vi "标样核查.vi"(11 "标样核查配置":T1={"数据保存间隔"=1.0, "水温标样值"=0.0, "pH标样值"=0.0, "溶解氧标样值"=0.0, "电导率标样值"=0.0, "浊度标样值"=0.0}) -> ()   [LabVIEW 2016, in "斯坦道多参数.lvlib"]
panel:
  out "运行状态":u16(ring) items=["空闲", "水样测试", "标样核查"]
  out "seconds since 1Jan1904":timestamp
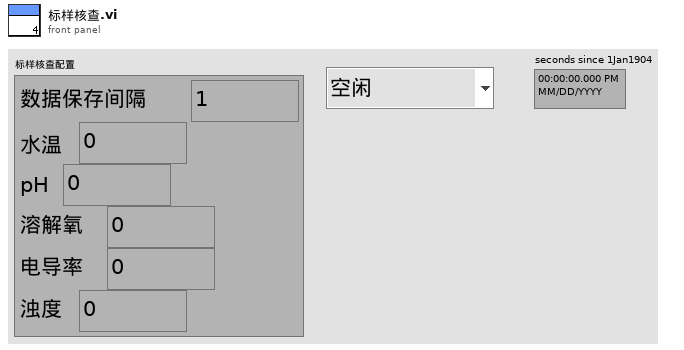
[diagram p1: front panel]
types:
  T1 = cluster{"数据保存间隔":dbl, "水温标样值":dbl, "pH标样值":dbl, "溶解氧标样值":dbl, "电导率标样值":dbl, "浊度标样值":dbl}
  T2 = cluster{"因子编码":string, "单位":string, "标样参考值":sgl, "水样数据时间":timestamp, "水样实测值":sgl, "水样数据标识":string, "探头温度":sgl}
  T3 = typedef "LVDateTimeRec.ctl" = cluster{"秒数的小数部分":dbl, "秒":i32, "分":i32, "时":i32, "日":i32, "月":i32, "年":i32, "天数（周）":i32, "天数（年）":i32, "DST":i32}
  T4 = cluster{"温度测量值":sgl, "DO%":sgl, "DOmg/L":sgl, "温度偏移修正值":sgl}
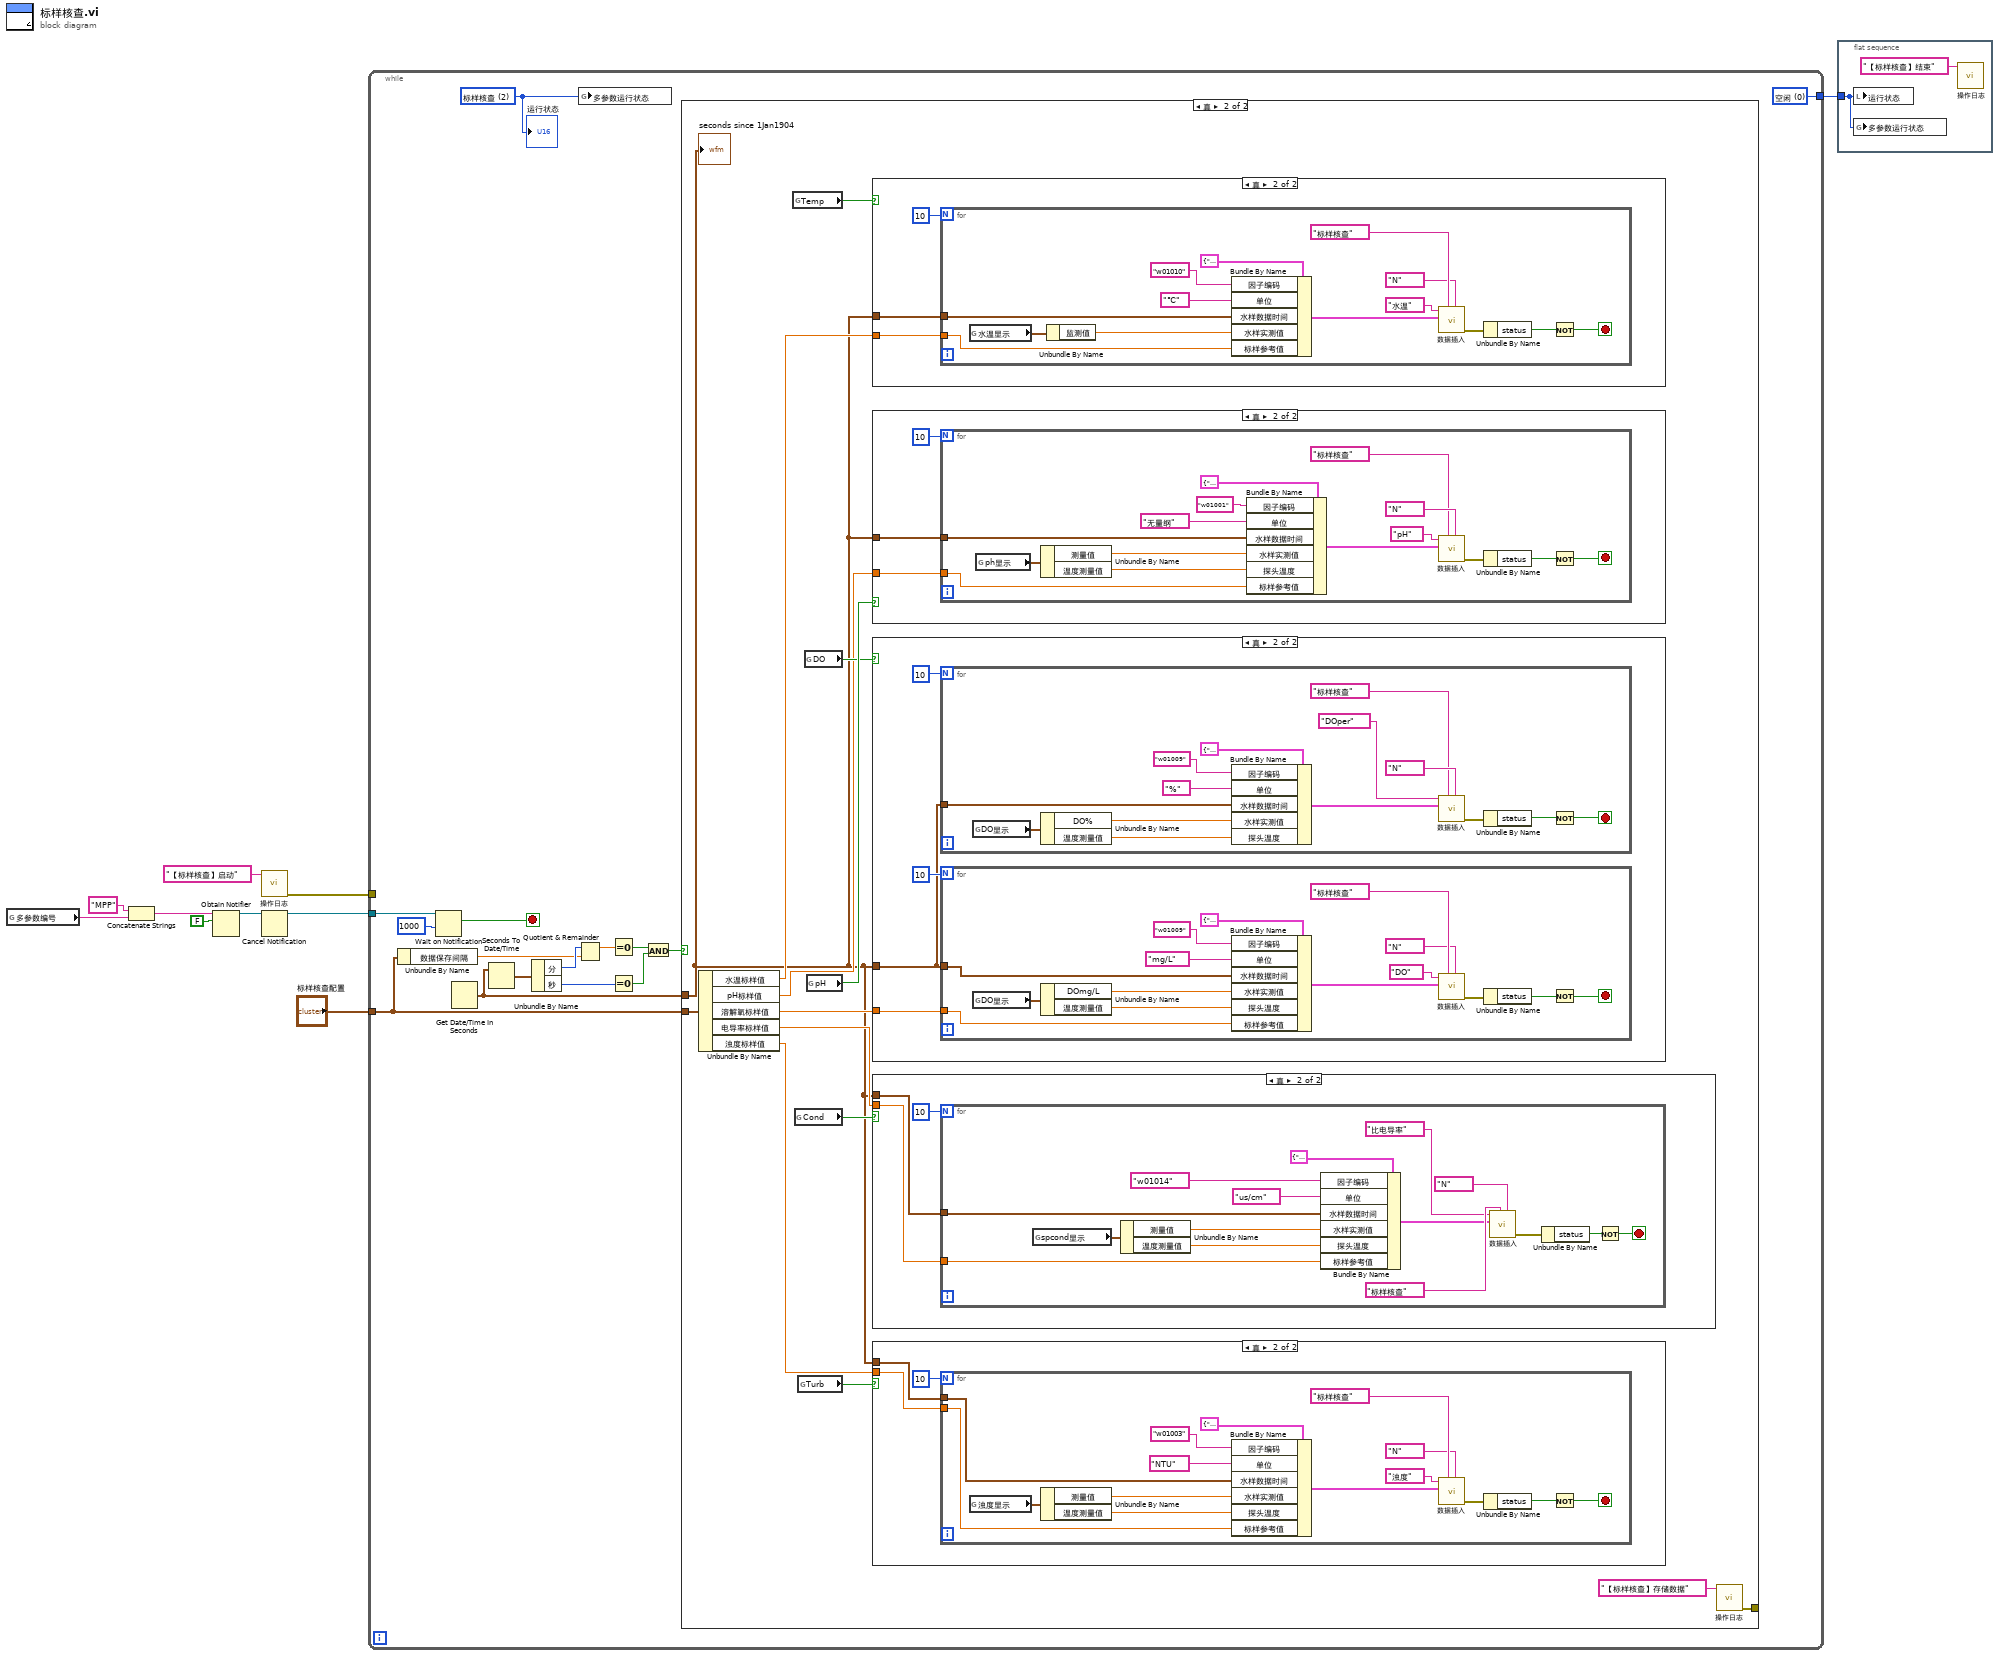
[diagram p0: block diagram]
diagram:
  n1 = global read "多参数全局变量.vi" "多参数编号"() -> (w3:string)
  n2 = Concatenate Strings("MPP" ("名称（未命名）"), w3) -> (w4:string)
  n3 = Obtain Notifier(name (unnamed)=w4, notification data type=FALSE) -> (notifier out=w7:refnum<notifier>)  [unwired: 2 in, 2 out]
  n4 = call "操作日志.vi"("日志信息"="【标样核查】启动") -> ("error out"=w1:errorcluster)  [unwired: 10 in]
  n5 = Cancel Notification(0:w7) -> (8:w6:refnum<notifier>)  [unwired: 1 in, 2 out]
  n6 = while {
    tunnel: "标样核查配置" -> [w21]
    tunnel: [w15] -> w5
    tunnel: w6 -> [w14]
    tunnel: w1 -> [_]
    stop <- w12 stop-if-true
    w15 = u16 0 items=["空闲", "水样测试", "标样核查"] ("多参数运行状态")
    w11 = u16 2 items=["空闲", "水样测试", "标样核查"] ("多参数运行状态")
    n7 = Unbundle By Name(w21) -> ("数据保存间隔"=w19:dbl)
    n8 = Wait on Notification(notifier=w14, timeout in ms (-1)=1000 ("超时毫秒(-1)")) -> (notification=w12:bool)  [unwired: 2 in, 3 out]
    n9 = Get Date/Time In Seconds() -> (seconds since 1Jan1904=w16:timestamp)
    n10 = Seconds To Date/Time(time stamp (now)=w16) -> (date time rec=w25:T3)  [unwired: 1 in]
    n11 = Unbundle By Name(w25) -> ("分"=w20:i32, "秒"=w24:i32)
    n12 = Quotient & Remainder(x=w20, y=w19) -> (x-y*floor(x/y)=w18:dbl)  [unwired: 1 out]
    n13 = global write "多参数全局变量.vi" "多参数运行状态"(w11) -> ()
    n14 = Equal To 0?(x=w18) -> (x = 0?=w17:bool)
    n15 = Equal To 0?(x=w24) -> (x = 0?=w23:bool)
    n16 = And(x=w17, y=w23) -> (x .and. y?=w22:bool)
    n17 = case shown="真" w22 {
      tunnel: w21 -> [_ w34]
      tunnel: w16 -> [_ w26]
      tunnel: [_ w27] -> _
      frame False {
      }
      frame True {
        n18 = Unbundle By Name(w34) -> ("水温标样值"=w33:dbl, "pH标样值"=w32:dbl, "溶解氧标样值"=w31:dbl, "电导率标样值"=w30:dbl, "浊度标样值"=w29:dbl)
        n19 = global read "断电保存变量.vi" "Temp"() -> (w39:bool)
        n20 = global read "断电保存变量.vi" "Cond"() -> (w36:bool)
        n21 = global read "断电保存变量.vi" "Turb"() -> (w35:bool)
        n22 = global read "断电保存变量.vi" "DO"() -> (w37:bool)
        n23 = global read "断电保存变量.vi" "pH"() -> (w38:bool)
        n24 = case shown="真" w39 {
          tunnel: w33 -> [_ w129]
          tunnel: w26 -> [_ w128]
          frame False {
          }
          frame True {
            n25 = for {
              N: 10 -> [_]
              tunnel: w129 -> [w136]
              tunnel: w128 -> [w133]
              stop <- w130 stop-if-true
              n26 = global read "多参数全局变量.vi" "水温显示"() -> (w135:cluster{"CH":u16, "监测值":dbl, "温度偏移修正值":sgl})
              n27 = Unbundle By Name(w135) -> ("监测值"=w134:dbl)
              n28 = Bundle By Name(cluster=T2 {"因子编码"="w01003", "单位"="无量纲", "标样参考值"=0.0, "水样数据时间"=timestamp(0 s since 1904-01-01), "水样实测值"=0.0, "水样数据标识"="N", "探头温度"=0.0} ("data in"), "因子编码"="w01010", "单位"="℃", "水样数据时间"=w133, "水样实测值"=w134, "标样参考值"=w136) -> (w142:T2)
              n29 = call "数据插入.vi"("数据标记表"="N", "测量模式"="标样核查", "data in"=w142, "table输入"="水温") -> ("error out"=w132:errorcluster)  [unwired: 7 in]
              n30 = Unbundle By Name(w132) -> ("status"=w131:bool)
              n31 = Not(x=w131) -> (.not. x?=w130:bool)
            }
          }
        }
        n32 = case shown="真" w38 {
          tunnel: w32 -> [_ w111]
          tunnel: w26 -> [_ w109]
          frame False {
          }
          frame True {
            n33 = for {
              N: 10 -> [_]
              tunnel: w111 -> [w119]
              tunnel: w109 -> [w112]
              stop <- w113 stop-if-true
              n34 = global read "多参数全局变量.vi" "ph显示"() -> (w118:cluster{"温度测量值":sgl, "测量值":sgl, "温度偏移修正值":sgl})
              n35 = Unbundle By Name(w118) -> ("测量值"=w117:sgl, "温度测量值"=w116:sgl)
              n36 = Bundle By Name(cluster=T2 {"因子编码"="w01003", "单位"="无量纲", "标样参考值"=0.0, "水样数据时间"=timestamp(0 s since 1904-01-01), "水样实测值"=0.0, "水样数据标识"="N", "探头温度"=0.0} ("data in"), "因子编码"="w01001", "单位"="无量纲", "水样数据时间"=w112, "水样实测值"=w117, "探头温度"=w116, "标样参考值"=w119) -> (w124:T2)
              n37 = call "数据插入.vi"("数据标记表"="N", "测量模式"="标样核查", "data in"=w124, "table输入"="pH") -> ("error out"=w115:errorcluster)  [unwired: 7 in]
              n38 = Unbundle By Name(w115) -> ("status"=w114:bool)
              n39 = Not(x=w114) -> (.not. x?=w113:bool)
            }
          }
        }
        n40 = case shown="真" w37 {
          tunnel: w31 -> [_ w79]
          tunnel: w26 -> [_ w76]
          frame False {
          }
          frame True {
            n41 = for {
              N: 10 -> [_]
              tunnel: w76 -> [w80]
              stop <- w81 stop-if-true
              n42 = global read "多参数全局变量.vi" "DO显示"() -> (w84:T4)
              n43 = Unbundle By Name(w84) -> ("DO%"=w88:sgl, "温度测量值"=w86:sgl)
              n44 = Bundle By Name(cluster=T2 {"因子编码"="w01003", "单位"="无量纲", "标样参考值"=0.0, "水样数据时间"=timestamp(0 s since 1904-01-01), "水样实测值"=0.0, "水样数据标识"="N", "探头温度"=0.0} ("data in"), "因子编码"="w01009", "单位"="%", "水样数据时间"=w80, "水样实测值"=w88, "探头温度"=w86) -> (w85:T2)
              n45 = call "数据插入.vi"("数据标记表"="N", "测量模式"="标样核查", "data in"=w85, "table输入"="DOper") -> ("error out"=w83:errorcluster)  [unwired: 7 in]
              n46 = Unbundle By Name(w83) -> ("status"=w82:bool)
              n47 = Not(x=w82) -> (.not. x?=w81:bool)
            }
            n48 = for {
              N: 10 -> [_]
              tunnel: w79 -> [w99]
              tunnel: w76 -> [w94]
              stop <- w95 stop-if-true
              n49 = global read "多参数全局变量.vi" "DO显示"() -> (w98:T4)
              n50 = Unbundle By Name(w98) -> ("DOmg/L"=w106:sgl, "温度测量值"=w108:sgl)
              n51 = Bundle By Name(cluster=T2 {"因子编码"="w01003", "单位"="无量纲", "标样参考值"=0.0, "水样数据时间"=timestamp(0 s since 1904-01-01), "水样实测值"=0.0, "水样数据标识"="N", "探头温度"=0.0} ("data in"), "因子编码"="w01009", "单位"="mg/L", "水样数据时间"=w94, "水样实测值"=w106, "探头温度"=w108, "标样参考值"=w99) -> (w105:T2)
              n52 = call "数据插入.vi"("数据标记表"="N", "测量模式"="标样核查", "data in"=w105, "table输入"="DO") -> ("error out"=w97:errorcluster)  [unwired: 7 in]
              n53 = Unbundle By Name(w97) -> ("status"=w96:bool)
              n54 = Not(x=w96) -> (.not. x?=w95:bool)
            }
          }
        }
        n55 = case shown="真" w36 {
          tunnel: w30 -> [_ w60]
          tunnel: w26 -> [_ w58]
          frame False {
          }
          frame True {
            n56 = for {
              N: 10 -> [_]
              tunnel: w60 -> [w68]
              tunnel: w58 -> [w61]
              stop <- w62 stop-if-true
              n57 = global read "多参数全局变量.vi" "spcond显示"() -> (w67:cluster{"温度测量值":sgl, "测量值":sgl, "温度偏移修正值":sgl})
              n58 = Unbundle By Name(w67) -> ("测量值"=w66:sgl, "温度测量值"=w65:sgl)
              n59 = Bundle By Name(cluster=T2 {"因子编码"="w01003", "单位"="无量纲", "标样参考值"=0.0, "水样数据时间"=timestamp(0 s since 1904-01-01), "水样实测值"=0.0, "水样数据标识"="N", "探头温度"=0.0} ("data in"), "因子编码"="w01014", "单位"="us/cm", "水样数据时间"=w61, "水样实测值"=w66, "探头温度"=w65, "标样参考值"=w68) -> (w73:T2)
              n60 = call "数据插入.vi"("数据标记表"="N", "测量模式"="标样核查", "data in"=w73, "table输入"="比电导率") -> ("error out"=w64:errorcluster)  [unwired: 7 in]
              n61 = Unbundle By Name(w64) -> ("status"=w63:bool)
              n62 = Not(x=w63) -> (.not. x?=w62:bool)
            }
          }
        }
        n63 = case shown="真" w35 {
          tunnel: w29 -> [_ w42]
          tunnel: w26 -> [_ w40]
          frame False {
          }
          frame True {
            n64 = for {
              N: 10 -> [_]
              tunnel: w42 -> [w50]
              tunnel: w40 -> [w43]
              stop <- w44 stop-if-true
              n65 = global read "多参数全局变量.vi" "浊度显示"() -> (w49:cluster{"温度测量值":sgl, "测量值":sgl, "温度偏移修正值":sgl})
              n66 = Unbundle By Name(w49) -> ("测量值"=w48:sgl, "温度测量值"=w47:sgl)
              n67 = Bundle By Name(cluster=T2 {"因子编码"="w01003", "单位"="无量纲", "标样参考值"=0.0, "水样数据时间"=timestamp(0 s since 1904-01-01), "水样实测值"=0.0, "水样数据标识"="N", "探头温度"=0.0} ("data in"), "因子编码"="w01003", "单位"="NTU", "水样数据时间"=w43, "水样实测值"=w48, "探头温度"=w47, "标样参考值"=w50) -> (w56:T2)
              n68 = call "数据插入.vi"("数据标记表"="N", "测量模式"="标样核查", "data in"=w56, "table输入"="浊度") -> ("error out"=w46:errorcluster)  [unwired: 7 in]
              n69 = Unbundle By Name(w46) -> ("status"=w45:bool)
              n70 = Not(x=w45) -> (.not. x?=w44:bool)
            }
          }
        }
        n71 = call "操作日志.vi"("日志信息"="【标样核查】存储数据") -> ("error out"=w27:errorcluster)  [unwired: 10 in]
        "seconds since 1Jan1904" <- w26
      }
    }
    "运行状态" <- w11
  }
  n72 = flat-sequence {
    tunnel: w5 -> [w145]
    frame #0 {
      n73 = local write "运行状态"(w145) -> ()
      n74 = global write "多参数全局变量.vi" "多参数运行状态"(w145) -> ()
      n75 = call "操作日志.vi"("日志信息"="【标样核查】结束") -> ()  [unwired: 10 in, 1 out]
    }
  }
